vi "OpenCVdemo.vi"() -> ()   [LabVIEW 2018]
uses:
  <vilib>/picture/picture.llb/Draw True-Color Pixmap.vi
  OpenCVcamLV/OpenCVcamLV.lvlib
panel:
  out "FPS":dbl
  out "Frame":i32
  in  "Stop Button":bool
  out "2D Picture":picture
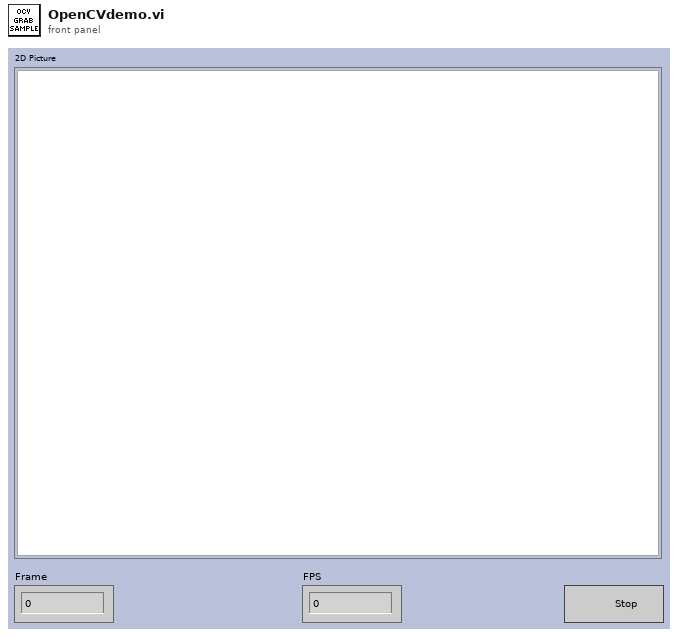
[diagram p1: front panel]
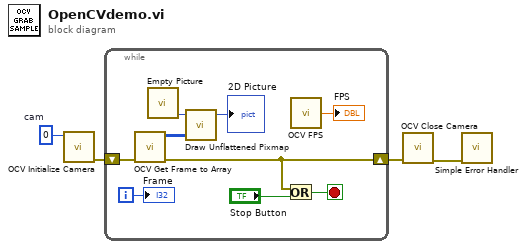
[diagram p0: block diagram]
diagram:
  w4 = 0  # cam
  n1 = call "OCV Initialize Camera.vi"("cam"=w4) -> ("error out"=w2:errorcluster)  [unwired: 10 in]
  n2 = while {
    shift-right: [w5] -> w3
    shift-left: w2 -> [w7]
    i -> [w10]
    stop <- w6 stop-if-true
    n3 = call "OCV Get Frame to Array.vi"("error in (no error)"=w7) -> ("error out"=w5:errorcluster, "frame"=w9:u32[][])  [unwired: 9 in]
    n4 = call "Empty Picture"() -> ("empty picture"=w12:picture)
    n5 = call-poly <vilib>:"Draw Unflattened Pixmap.vi"("picture"=w12, "data (RGB format)"=w9) -> ("new picture"=→"2D Picture":picture)  [unwired: 7 in]
    n6 = Or(x=w5, y="Stop Button") -> (x .or. y?=w6:bool)
    n7 = call "OCV FPS.vi"() -> ("FPS"=→"FPS":dbl)  [unwired: 3 in, 1 out]
    "Frame" <- w10
  }
  n8 = call "OCV Close Camera.vi"("error in (no error)"=w3) -> ("error out"=w1:errorcluster)  [unwired: 10 in]
  n9 = call <vilib>:"Simple Error Handler.vi"("error in (no error)"=w1) -> ()  [unwired: 4 in, 5 out]
